vi "AbortTrial.vi"(8 "error in (no error)":errorcluster, 10 "AbortReason":string, 11 "TrialBasedExperiment in":refnum<class "MatlabExperiment.lvclass">) -> (0 "error out":errorcluster, 3 "TrialBasedExperiment out":refnum<class "MatlabExperiment.lvclass">)   [LabVIEW 2014, in "AcquisitionCoreObjects.lvlib" / "MatlabExperiment.lvclass"]
uses:
  MatlabExperiment.lvclass
  TrialBasedExperimentObject/TrialBasedExperiment.lvclass
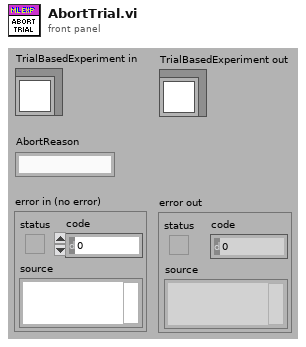
[diagram p1: front panel]
types:
  T1 = cluster{"Variable name":string, "AbortReason":string}
  T2 = cluster{"Variable name":string, "AbortReason":string}[]
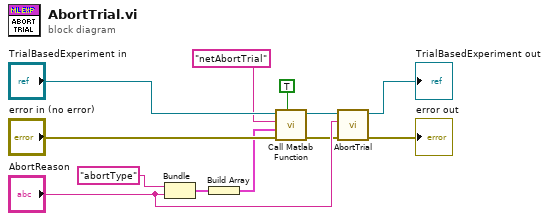
[diagram p0: block diagram]
diagram:
  n1 = Bundle("Variable name"="abortType", "AbortReason"="AbortReason") -> (w7:T1)  [unwired: 1 out]
  n2 = Build Array(w7) -> (w6:T2)
  n3 = call-dynamic "Call Matlab Function.vi"("Timestamp"=TRUE, "error in (no error)"="error in (no error)", "Matlab Param Array"=w6, "Function name"="netAbortTrial", "TrialBasedExperiment in"="TrialBasedExperiment in") -> ("error out"=w3:errorcluster, "TrialBasedExperiment out"=w4:refnum<class "MatlabExperiment.lvclass">)  [unwired: 3 in, 2 out]
  n4 = call-parent "AbortTrial.vi"("error in (no error)"=w3, "AbortReason"="AbortReason", "TrialBasedExperiment in"=w4) -> ("error out"=→"error out":errorcluster, "TrialBasedExperiment out"=→"TrialBasedExperiment out":refnum<class "MatlabExperiment.lvclass">)  [unwired: 7 in]
